vi "LS340_ReadChannel.vi"(6 "error in (no error)":errorcluster, 8 "Input (0: A)":u16(ring) items=["A", "B", "C", "D"], 9 "VISA resource name":refnum<visa-resource-name>) -> (0 "error out":errorcluster, 1 "Sensor Units Reading":dbl min=-7.5 max=300000.0 step=1e-05 format="%^.5e", 3 "VISA  out":refnum<visa-resource-name>, 4 "Kelvin Reading":dbl min=0.0 max=1645.0 step=1e-05 format="%^.5e", 5 "Celsius Reading":dbl min=-273.16 max=1372.0 step=1e-05 format="%^.5e")   [LabVIEW 2012]
doc: "This VI was designed to demonstrate typical usage of sub vi's containing the more common 340 functions.\n\nThis example configures the loop and setpoint of the instrument, allows for a delay, and then reads sensor and heater output data. The user is given the option of just reading data and not configuring the instrument."
uses:
  <instrlib>/Lake Shore Cryotronics 340/Lake Shore Cryotronics 340.lvlib
panel:
  # "Copyright 2005. National Instruments Corporation"
  # "340 Temperature Controller"
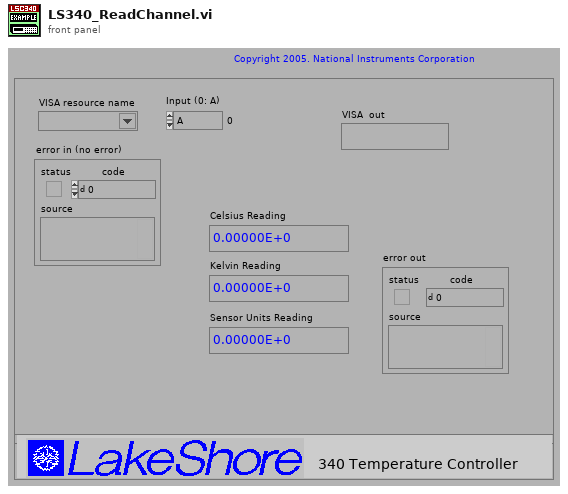
[diagram p1: front panel]
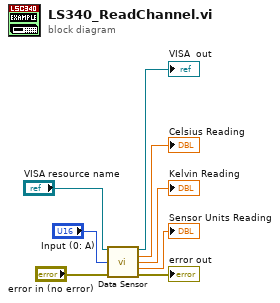
[diagram p0: block diagram]
diagram:
  n1 = call <instrlib>:"Data Sensor.vi"("VISA resource name"="VISA resource name", "Input (0: A)"="Input (0: A)", "error in (no error)"="error in (no error)") -> ("VISA resource name out"=→"VISA  out":refnum<visa-resource-name>, "Celsius Reading"=→"Celsius Reading":dbl, "Kelvin Reading"=→"Kelvin Reading":dbl, "Sensor Units Reading"=→"Sensor Units Reading":dbl, "error out"=→"error out":errorcluster)  [unwired: 8 in]
